vi "05 Graphs.vi"() -> ()   [LabVIEW 2019]
uses:
  _Subs/OpenDiagram/Open_XControl.xctl
panel:
  in  "OpenDiag":refnum<vi>(xcontrol)
  out "Waveform Graph 2":cluster{i32, dbl, i32[]}(graph)
  out "XY Graph 2":cluster{i32, dbl}[](graph)
  out "XY Graph":cluster{"X":i32[], dbl[]}(graph)
  out "Waveform Graph":i32[](graph)
  # "05 Graphs\nThis code compares some of the different ways to feed generated data to graphs \n\nInstructions:\n1. Hit the Run arrow to see the data being plotted.\n2. Analyze the block diagram and compare how data is formatted and plotted.\n3. Right click on any graph and go to Properties. Explore how you can modify the graph."
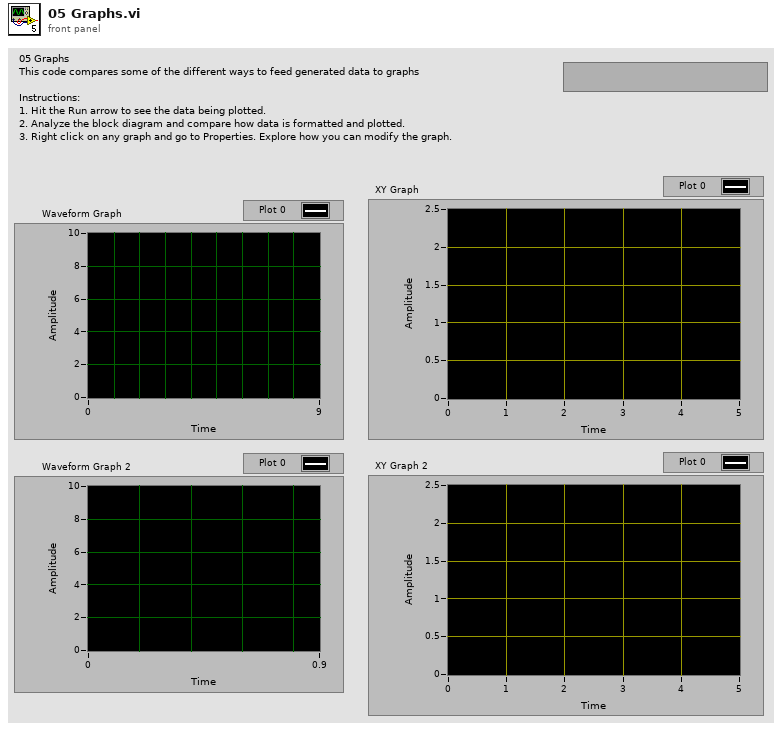
[diagram p1: front panel]
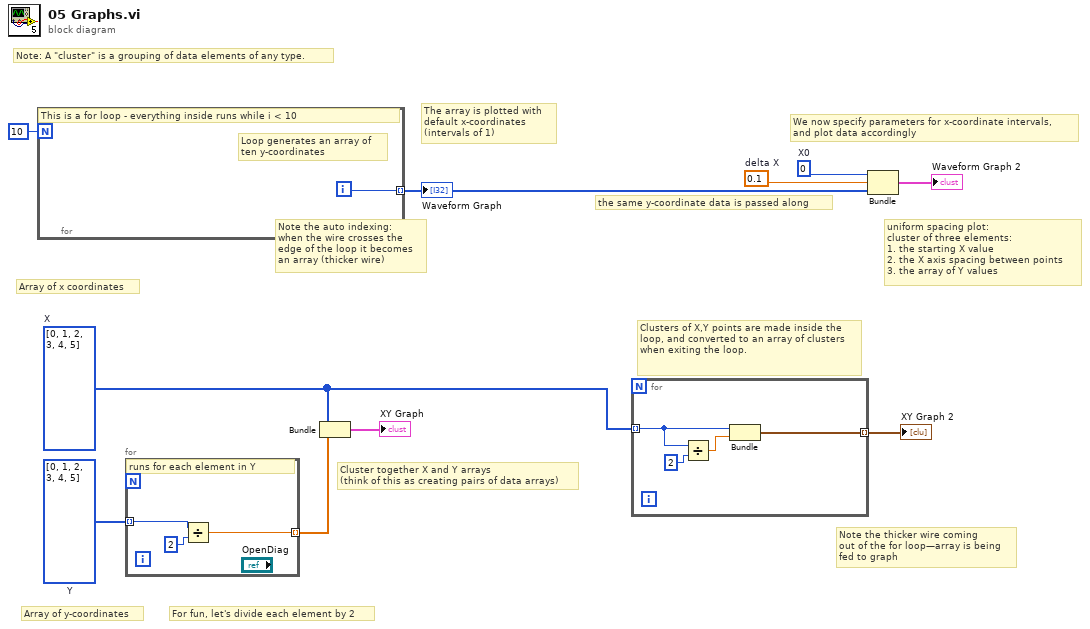
[diagram p0: block diagram]
diagram:
  w2 = 0.1  # delta X
  w3 = 0  # X0
  w9 = i32[] [0, 1, 2, 3, 4, 5]  # Y
  w6 = i32[] [0, 1, 2, 3, 4, 5]  # X
  # "Clusters of X,Y points are made inside the loop, and converted to an array of clusters when exiting the loop."
  # "Note: A \"cluster\" is a grouping of data elements of any type."
  # "For fun, let's divide each element by 2"
  # "Array of y-coordinates"
  # "We now specify parameters for x-coordinate intervals,\nand plot data accordingly"
  # "the same y-coordinate data is passed along"
  # "The array is plotted with \ndefault x-coordinates \n(intervals of 1)"
  # "Array of x coordinates"
  # "uniform spacing plot:\ncluster of three elements:\n1. the starting X value\n2. the X axis spacing between points\n3. the array of Y values"
  # "Note the thicker wire coming\nout of the for loop—array is being\nfed to graph"
  # "Cluster together X and Y arrays\n(think of this as creating pairs of data arrays)"
  # "Note the auto indexing:\nwhen the wire crosses the\nedge of the loop it becomes\nan array (thicker wire)"
  n1 = for {
    N: 10 -> [_]
    tunnel: [w11] -> w4 mode=indexing
    i -> [w11]
    # "Loop generates an array of \nten y-coordinates"
    # "This is a for loop - everything inside runs while i < 10"
  }
  "Waveform Graph" <- w4
  n2 = for {
    tunnel: w9 -> [w14] mode=indexing
    tunnel: [w12] -> w8 mode=indexing
    # "runs for each element in Y"
    n3 = Divide(x=w14, y=2) -> (x/y=w12:dbl)
  }
  n4 = Bundle("X"=w6, w8) -> (→"XY Graph":cluster{"X":i32[], dbl[]})  [unwired: 1 in]
  n5 = for {
    tunnel: w6 -> [w16] mode=indexing
    tunnel: [w15] -> w5 mode=indexing
    n6 = Divide(x=w16, y=2) -> (x/y=w17:dbl)
    n7 = Bundle(w16, w17) -> (w15:cluster{i32, dbl})  [unwired: 1 in]
  }
  "XY Graph 2" <- w5
  n8 = Bundle("X0"=w3, "delta X"=w2, w4) -> (→"Waveform Graph 2":cluster{"X0":i32, "delta X":dbl, i32[]})  [unwired: 1 in]
